vi "USB2XXXIIC24C32.vi"() -> ()   [LabVIEW 2010]
panel:
  in  "pConfig":T1
  out "Read Data(Hex)":string
  in  "Read Data Count":i32=8
  in  "Reg Addr(Hex)":u16 format="%x"
  in  "Slave Addr(Hex)":i16=80 format="%x"
  in  "Write Data(Hex)":string="11 22 33 44 55 66 77 88"
  in  "Channel Index":i32(ring) items=["CH0", "CH1", "CH2", "CH3", "CH4", "CH5", "CH6", "CH7"]
  in  "Device Index":i32(ring) items=["0", "1", "2", "3", "4", "5"]
  out "Flag(T:Write;F:Read)":bool=TRUE
  in  "stop":bool
  in  "Read":bool
  in  "Write":bool
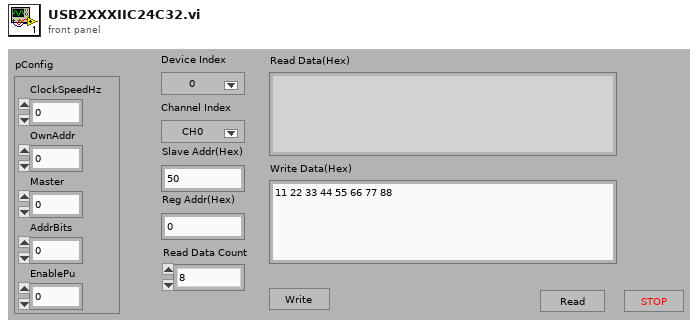
[diagram p1: front panel]
types:
  T1 = cluster{"ClockSpeedHz":u32, "OwnAddr":u16, "Master":u8, "AddrBits":u8, "EnablePu":u8}
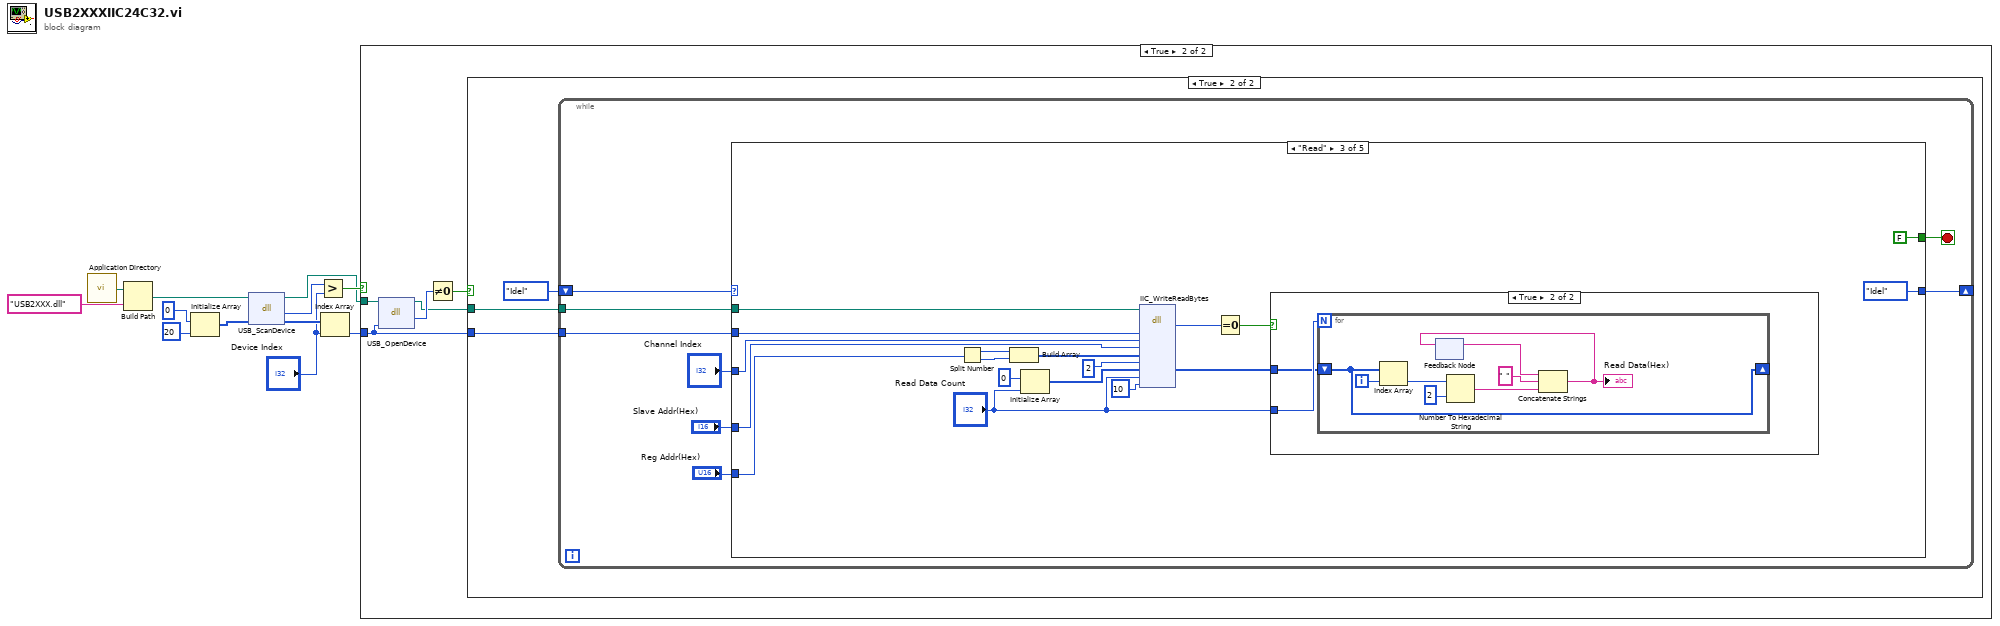
[diagram p0: block diagram]
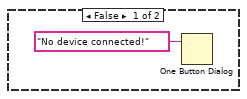
[diagram p2: hidden frame]
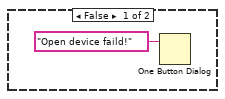
[diagram p3: hidden frame]
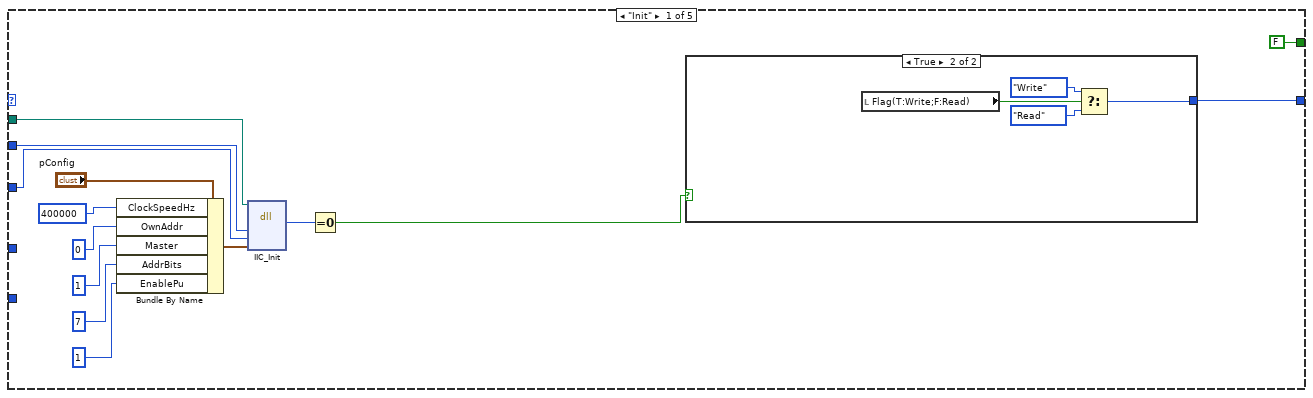
[diagram p4: hidden frame]
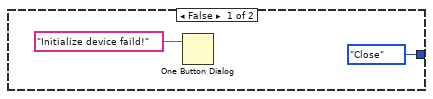
[diagram p5: hidden frame]
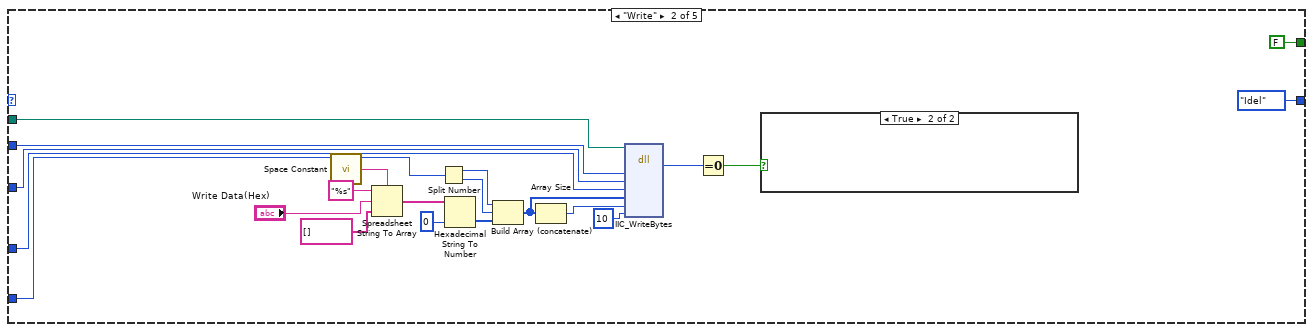
[diagram p6: hidden frame]
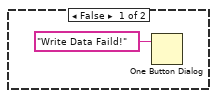
[diagram p7: hidden frame]
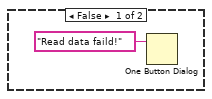
[diagram p8: hidden frame]
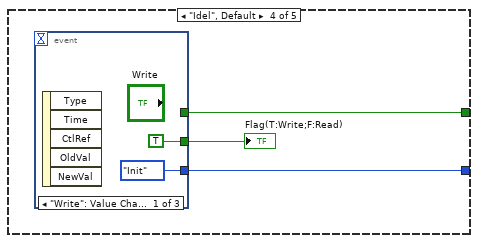
[diagram p9: hidden frame]
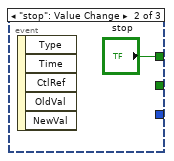
[diagram p10: hidden frame]
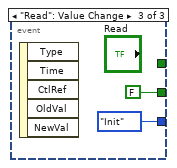
[diagram p11: hidden frame]
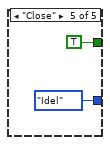
[diagram p12: hidden frame]
diagram:
  n1 = call <vilib>:"Application Directory.vi"() -> ("Application Directory"=w4:path)
  n2 = Build Path(base path=w4, name or relative path="USB2XXX.dll") -> (appended path=w3:path)
  n3 = Initialize Array(0, 20 ("dimension size")) -> (w9:i32[])
  n4 = dll-call lib="E:/Projects/USB2XXX_Example/sdk/api/Labview/USB2XXX.*" fn="USB_ScanDevice"(path in=w3, "pDevNum"=w9) -> (path out=w2:path, "return type"=w8:i32, "pDevNum"=w12:i32[])  [unwired: 2 in, 1 out]
  n5 = Greater?(x=w8, y="Device Index") -> (0:w7:bool)
  n6 = Index Array(array=w12, index="Device Index") -> (element=w6:i32)
  n7 = case shown="True" w7 {
    tunnel: w6 -> [_ w16]
    tunnel: w2 -> [_ w15]
    frame False {
      n8 = One Button Dialog(message="No device connected!") -> ()  [unwired: 1 in, 1 out]
    }
    frame True {
      n9 = dll-call lib="E:/Projects/USB2XXX_Example/sdk/api/Labview/USB2XXX.*" fn="USB_OpenDevice"(path in=w15, "DevIndex"=w16) -> (path out=w14:path, "return type"=w18:u8)  [unwired: 3 in, 1 out]
      n10 = Not Equal To 0?(x=w18) -> (x != 0?=w17:bool)
      n11 = case shown="True" w17 {
        tunnel: w16 -> [_ w21]
        tunnel: w14 -> [_ w20]
        frame False {
          n12 = One Button Dialog(message="Open device faild!") -> ()  [unwired: 1 in, 1 out]
        }
        frame True {
          n13 = while {
            shift-right: [w29] -> _
            shift-left: enum16{"Init", "Write", "Read", "Idel", "Close"}."Idel" ("Enum") -> [w30]
            tunnel: w21 -> [w24]
            tunnel: w20 -> [w23]
            stop <- w25 stop-if-true
            n14 = case shown="\"Read\"" w30 {
              tunnel: [w32 enum16{"Init", "Write", "Read", "Idel", "Close"}."Idel" ("Enum") enum16{"Init", "Write", "Read", "Idel", "Close"}."Idel" ("Enum") w102 enum16{"Init", "Write", "Read", "Idel", "Close"}."Idel" ("Enum")] -> w29
              tunnel: "Channel Index" -> [w34 w65 w85 _ _]
              tunnel: "Slave Addr(Hex)" -> [_ w59 w86 _ _]
              tunnel: "Reg Addr(Hex)" -> [_ w53 w76 _ _]
              tunnel: [FALSE FALSE FALSE w103 TRUE] -> w25
              tunnel: w24 -> [w33 w56 w78 _ _]
              tunnel: w23 -> [w31 w54 w77 _ _]
              frame "Init" {
                n15 = Bundle By Name(cluster="pConfig", "ClockSpeedHz"=u32 400000, "OwnAddr"=u16 0, "Master"=u8 1, "AddrBits"=u8 7, "EnablePu"=u8 1) -> (w42:T1)
                n16 = dll-call lib="E:/Projects/USB2XXX_Example/sdk/api/Labview/USB2XXX.*" fn="IIC_Init"(path in=w31, "DevIndex"=w33, "IICIndex"=w34, "pConfig"=w42) -> ("return type"=w36:i32)  [unwired: 5 in, 2 out]
                n17 = Equal To 0?(x=w36) -> (x = 0?=w35:bool)
                n18 = case shown="True" w35 {
                  tunnel: [enum16{"Init", "Write", "Read", "Idel", "Close"}."Close" ("Enum") w47] -> w32
                  frame False {
                    n19 = One Button Dialog(message="Initialize device faild!") -> ()  [unwired: 1 in, 1 out]
                  }
                  frame True {
                    n20 = local read "Flag(T:Write;F:Read)"() -> (w50:bool)
                    n21 = Select(t=enum16{"Init", "Write", "Read", "Idel", "Close"}."Write" ("Enum"), s=w50, f=enum16{"Init", "Write", "Read", "Idel", "Close"}."Read" ("Enum")) -> (s? t:f=w47:enum16{"Init", "Write", "Read", "Idel", "Close"})
                  }
                }
              }
              frame "Write" {
                n22 = call <vilib>:"Space Constant.vi"() -> ("String"=w67:string)
                n23 = Spreadsheet String To Array(delimiter (Tab)=w67, format string="%s", spreadsheet string="Write Data(Hex)", array type (2D Dbl)=string[] []) -> (array=w70:string[])
                n24 = Split Number(x=w53) -> (hi(x)=w51:u8, lo(x)=w52:u8)
                n25 = Hexadecimal String To Number(string=w70, default (0uL)=u8 0 ("default (0 U32)")) -> (number=w58:u8[])  [unwired: 1 in, 1 out]
                n26 = Build Array (concatenate)(w51, w52, w58) -> (w55:u8[])
                n27 = Array Size(array=w55) -> (size(s)=w64:i32)
                n28 = dll-call lib="E:/Projects/USB2XXX_Example/sdk/api/Labview/USB2XXX.*" fn="IIC_WriteBytes"(path in=w54, "DevIndex"=w56, "IICIndex"=w65, "SlaveAddr"=w59, "pWriteData"=w55, "WriteLen"=w64, "TimeOutMs"=10) -> ("return type"=w62:i32)  [unwired: 8 in, 2 out]
                n29 = Equal To 0?(x=w62) -> (x = 0?=w61:bool)
                n30 = case shown="True" w61 {
                  frame False {
                    n31 = One Button Dialog(message="Write Data Faild!") -> ()  [unwired: 1 in, 1 out]
                  }
                  frame True {
                  }
                }
              }
              frame "Read" {
                n32 = Split Number(x=w76) -> (hi(x)=w75:u8, lo(x)=w74:u8)
                n33 = Build Array(w75, w74) -> (w73:u8[])
                n34 = Initialize Array(u8 0 ("element"), "Read Data Count") -> (w88:u8[])
                n35 = dll-call lib="E:/Projects/USB2XXX_Example/sdk/api/Labview/USB2XXX.*" fn="IIC_WriteReadBytes"(path in=w77, "DevIndex"=w78, "IICIndex"=w85, "SlaveAddr"=w86, "pWriteData"=w73, "WriteLen"=2 ("dimension size"), "pReadData"=w88, "ReadLen"="Read Data Count", "TimeOutMs"=10) -> ("return type"=w84:i32, "pReadData"=w80:u8[])  [unwired: 9 in, 2 out]
                n36 = Equal To 0?(x=w84) -> (x = 0?=w83:bool)
                n37 = case shown="True" w83 {
                  tunnel: "Read Data Count" -> [_ w93]
                  tunnel: w80 -> [_ w92]
                  frame False {
                    n38 = One Button Dialog(message="Read data faild!") -> ()  [unwired: 1 in, 1 out]
                  }
                  frame True {
                    n39 = for {
                      N: w93 -> [_]
                      shift-right: [w94] -> _
                      shift-left: w92 -> [w94]
                      i -> [w101]
                      n40 = Index Array(array=w94, index=w101) -> (element=w100:u8)
                      n41 = feedback #1() -> (w98:string)  [unwired: 1 in]
                      n42 = Number To Hexadecimal String(1:i16 2 ("width (-)"), 2:w100) -> (0:w96:string)
                      n43 = Concatenate Strings(w98, " " ("string"), w96) -> (w95:string)
                      "Read Data(Hex)" <- w95
                      n44 = feedback-in #1(w95) -> ()
                    }
                  }
                }
              }
              frame "Idel", Default {
                n45 = event shown="[0] \"Write\": Value Change" {
                  selector: _ -> [_ _ _]
                  dyn-events: _ -> [_ _ _]
                  timeout: _ -> [_ _ _]
                  tunnel: [TRUE _ FALSE] -> w104
                  tunnel: [_ "stop" _] -> w103
                  tunnel: [enum16{"Init", "Write", "Read", "Idel", "Close"}."Init" ("Enum") _ enum16{"Init", "Write", "Read", "Idel", "Close"}."Init" ("Enum")] -> w102
                  event "Write": Value Change {
                    n46 = event-data() -> ()  [unwired: 1 in, 5 out]
                  }
                  event "stop": Value Change {
                    n47 = event-data() -> ()  [unwired: 1 in, 5 out]
                  }
                  event "Read": Value Change {
                    n48 = event-data() -> ()  [unwired: 1 in, 5 out]
                  }
                }
                "Flag(T:Write;F:Read)" <- w104
              }
              frame "Close" {
              }
            }
          }
        }
      }
    }
  }
